vi "Center Image In Rectangle.vi"(8 "Center Vertically? (True)":bool=TRUE, 9 "Background Color":u32(colorbox)=16777215, 10 "Rectangle":T1={"Width"=350, "Height"=350}, 11 "Picture In":picture) -> (3 "Picture Out (Centered)":picture)   [LabVIEW 2016]
uses:
  <vilib>/Utility/miscctls.llb/LVBoundsTypeDef.ctl
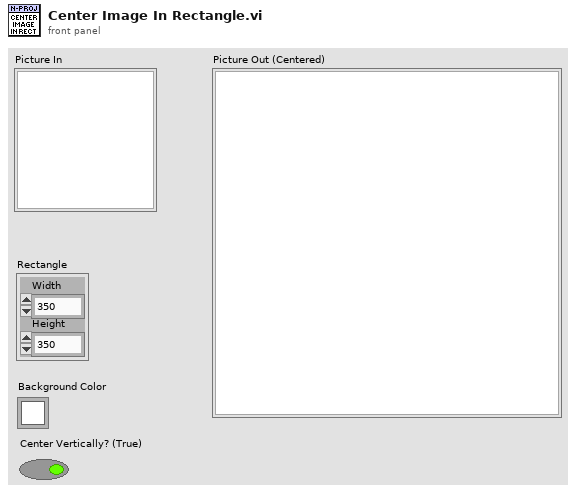
[diagram p1: front panel]
types:
  T1 = typedef "LVBoundsTypeDef.ctl" = cluster{"Width":u32, "Height":u32}
  T2 = typedef "imagedata.ctl" = cluster{"image type":i32, "image depth":i32, "image":u8[], "mask":u8[], "colors":u32[], "Rectangle":cluster{"left":i16, "top":i16, "right":i16, "bottom":i16}}
  T3 = cluster{"left":i16, "top":i16, "right":i16, "bottom":i16}
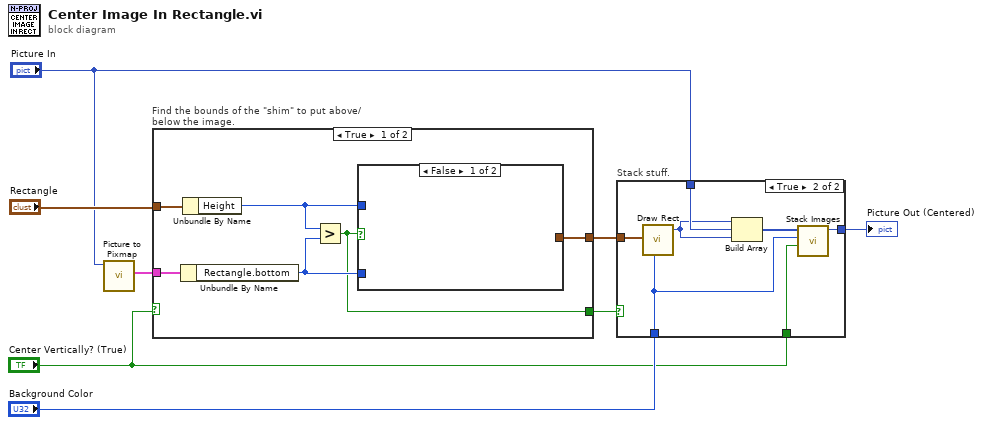
[diagram p0: block diagram]
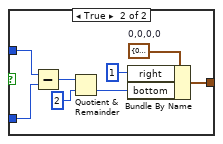
[diagram p3: hidden frame]
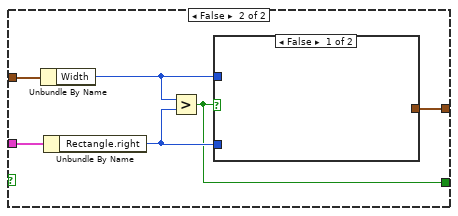
[diagram p4: hidden frame]
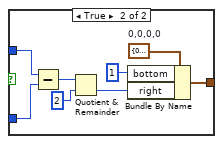
[diagram p5: hidden frame]
diagram:
  n1 = call <vilib>:"Picture to Pixmap.vi"("picture"="Picture In") -> ("image data"=w7:T2)  [unwired: 9 in, 1 out]
  n2 = case "Find the bounds of the \"shim\" to put above/below the image." shown="True" "Center Vertically? (True)" {
    tunnel: "Rectangle" -> [w14 w28]
    tunnel: w7 -> [w13 w27]
    tunnel: [w10 w24] -> w5
    tunnel: [w9 w23] -> w1
    frame True {
      n3 = Unbundle By Name(w13) -> ("Rectangle.bottom"=w12:i16)
      n4 = Unbundle By Name(w14) -> ("Height"=w11:u32)
      n5 = Greater?(x=w11, y=w12) -> (0:w9:bool)
      n6 = case shown="False" w9 {
        tunnel: w12 -> [_ w21]
        tunnel: w11 -> [_ w22]
        tunnel: [_ w16] -> w10
        frame False {
        }
        frame True {
          w15 = T3 {"left"=0, "top"=0, "right"=0, "bottom"=0}  # 0,0,0,0
          n7 = Subtract(x=w22, y=w21) -> (x-y=w20:u32)
          n8 = Quotient & Remainder(x=w20, y=u32 2) -> (floor(x/y)=w17:u32)  [unwired: 1 out]
          n9 = Bundle By Name(cluster=w15, "right"=i16 1 ("bottom"), "bottom"=w17) -> (w16:T3)
        }
      }
    }
    frame False {
      n10 = Unbundle By Name(w28) -> ("Width"=w25:u32)
      n11 = Unbundle By Name(w27) -> ("Rectangle.right"=w26:i16)
      n12 = Greater?(x=w25, y=w26) -> (0:w23:bool)
      n13 = case shown="False" w23 {
        tunnel: w26 -> [_ w35]
        tunnel: w25 -> [_ w36]
        tunnel: [_ w30] -> w24
        frame False {
        }
        frame True {
          w29 = T3 {"left"=0, "top"=0, "right"=0, "bottom"=0}  # 0,0,0,0
          n14 = Subtract(x=w36, y=w35) -> (x-y=w34:u32)
          n15 = Quotient & Remainder(x=w34, y=u32 2) -> (floor(x/y)=w31:u32)  [unwired: 1 out]
          n16 = Bundle By Name(cluster=w29, "bottom"=i16 1, "right"=w31) -> (w30:T3)
        }
      }
    }
  }
  n17 = case "Stack stuff." shown="True" w1 {
    tunnel: [w37 w44] -> w6
    tunnel: w5 -> [_ w43]
    tunnel: "Picture In" -> [w37 w42]
    tunnel: "Background Color" -> [_ w38]
    tunnel: "Center Vertically? (True)" -> [_ w39]
    frame False {
    }
    frame True {
      n18 = call <vilib>:"Draw Rect.vi"("rect"=w43, "color(black)"=w38) -> ("new picture"=w41:picture)  [unwired: 7 in]
      n19 = Build Array(w41, w42, w41) -> (w40:picture[])
      n20 = call <resource>:"Stack Images.vi"("Vertical?"=w39, "BG Color"=w38, "Array"=w40) -> ("empty picture"=w44:picture)  [unwired: 8 in]
    }
  }
  "Picture Out (Centered)" <- w6
